vi "Tabulate TDMS Name Mapping.vi"(8 "error in":errorcluster, 11 "measurement configuration":T1={"TDMS File Path"="", "TDMS Channels"=["Chn0"], "FGEN Resource Names"=[], "TDMS Groups"=[], "FGEN Waveform Names"=[], "Waveform Sequence"=["Wfm1"], "Loops Sequence"=[], "Markers Sequence"=[]}) -> (0 "error out":errorcluster, 3 "TDMS Name Mapping":T2)   [LabVIEW 2025, in "FGEN Arb Sequence Mode.lvclass"]
uses:
  FGEN Arb Sequence Mode.lvclass
  Measurement Configuration.ctl
  67890edf-85c8-4520-b9a4-a1863d36d414.vi
  00e03d3f-0884-43fe-8b00-c6cbeff4e0a9.vi
  5d0afab6-27d8-4637-a328-ab46698b29a4.vi
  <vilib>/Utility/error.llb/Error Cluster From Error Code.vi
  <vilib>/ErrorRing/Error Ring.xnode
  FGEN Arb Sequence Mode.lvclass/FGEN Arb Sequence Mode.ctl
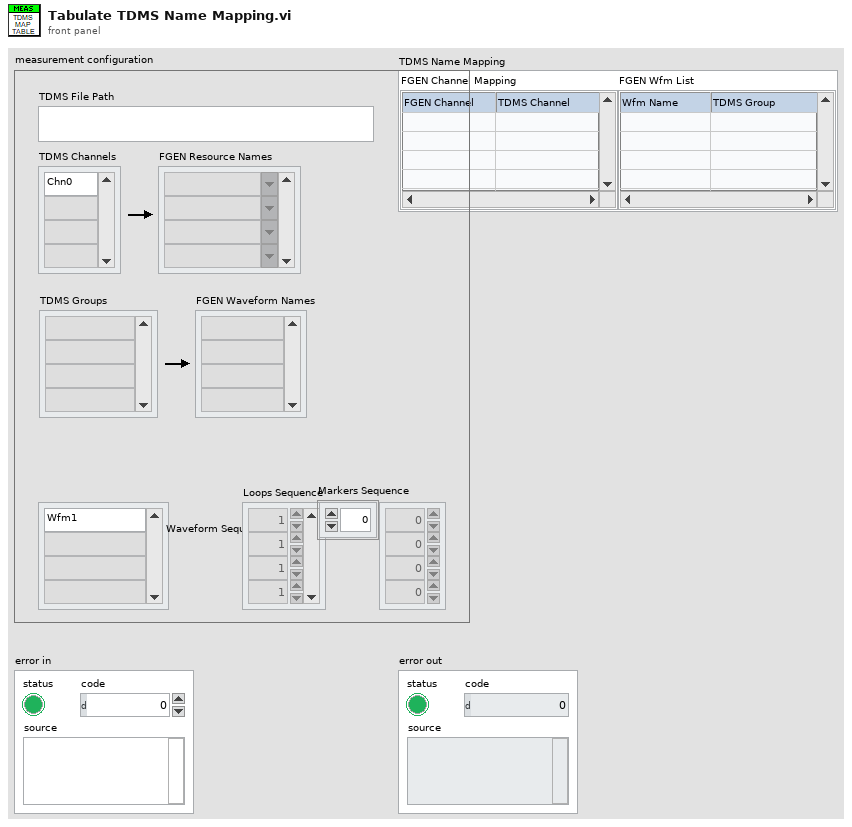
[diagram p1: front panel]
types:
  T1 = typedef "FGEN Arb Sequence Mode.lvclass/Measurement Configuration.ctl" = cluster{"TDMS File Path":string, "TDMS Channels":string[], "FGEN Resource Names":string[], "TDMS Groups":string[], "FGEN Waveform Names":string[], "Waveform Sequence":string[], "Loops Sequence":u32[], "Markers Sequence":i32[]}
  T2 = cluster{"FGEN Channel Mapping":string[][], "FGEN Wfm List":string[][]}
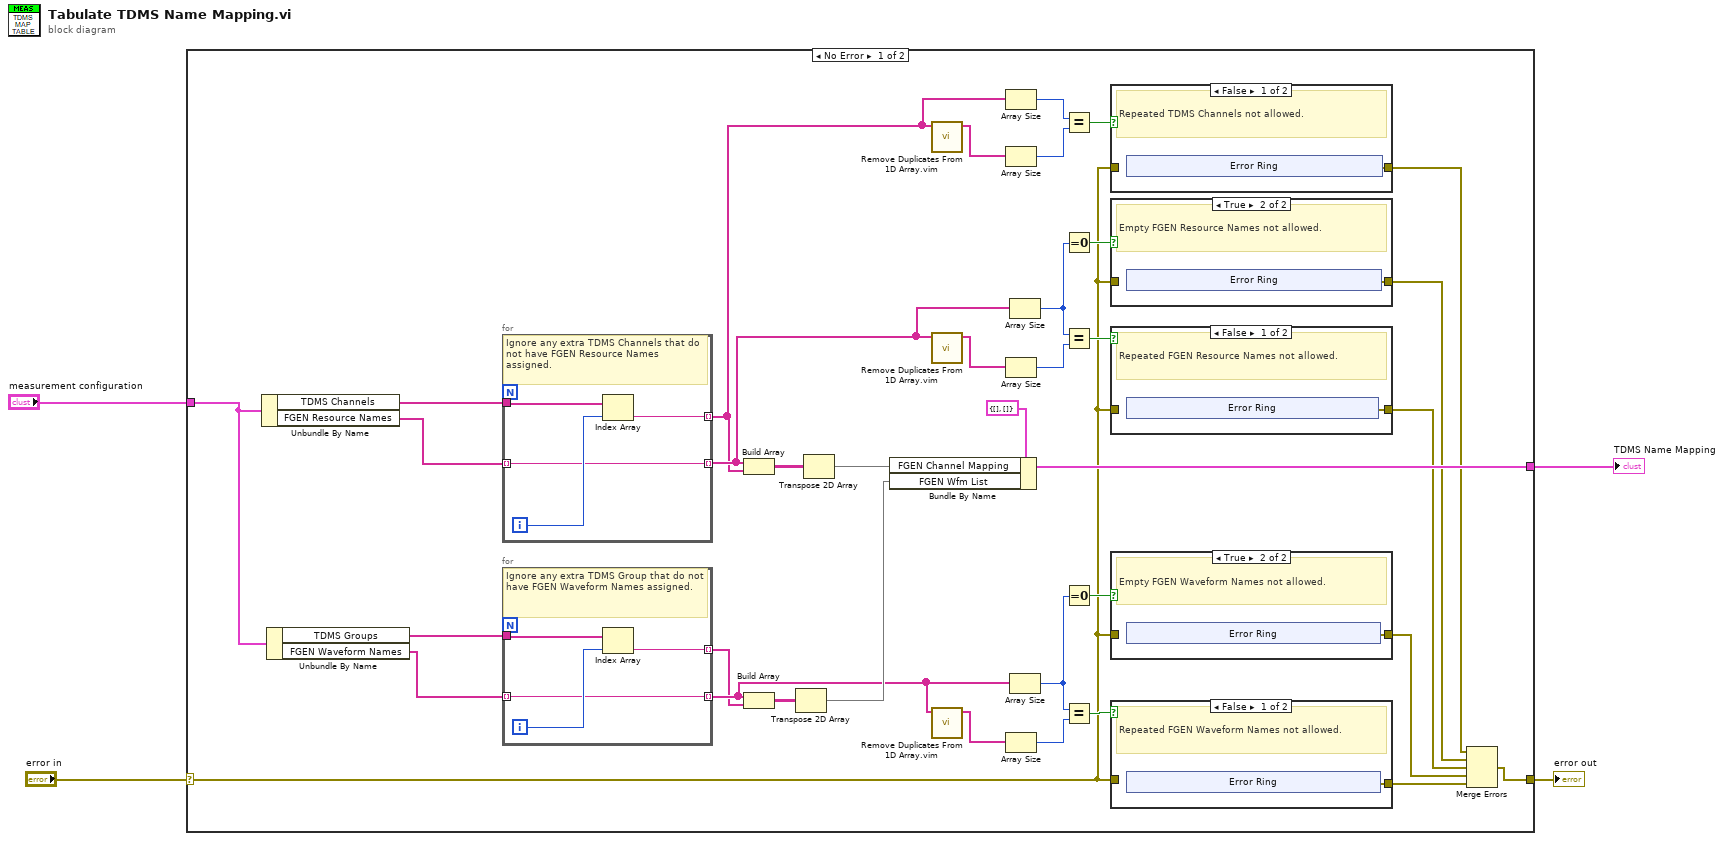
[diagram p0: block diagram]
diagram:
  n1 = case shown="No Error" "error in" {
    selector: "error in" -> [w5 w84]
    tunnel: [w26 w84] -> w3
    tunnel: "measurement configuration" -> [w40 _]
    tunnel: [w37 _] -> w1
    frame No Error {
      n2 = Unbundle By Name(w40) -> ("TDMS Channels"=w13:string[], "FGEN Resource Names"=w39:string[])
      n3 = Unbundle By Name(w40) -> ("TDMS Groups"=w9:string[], "FGEN Waveform Names"=w35:string[])
      n4 = for {
        tunnel: w39 -> [w63] mode=indexing
        tunnel: w13 -> [w65]
        tunnel: [w63] -> w29 mode=indexing
        tunnel: [w62] -> w7 mode=indexing
        i -> [w64]
        # "Ignore any extra TDMS Channels that do not have FGEN Resource Names assigned."
        n5 = Index Array(array=w65, index=w64) -> (element=w62:string)
      }
      n6 = for {
        tunnel: w35 -> [w81] mode=indexing
        tunnel: w9 -> [w83]
        tunnel: [w81] -> w22 mode=indexing
        tunnel: [w80] -> w8 mode=indexing
        i -> [w82]
        # "Ignore any extra TDMS Group that do not have FGEN Waveform Names assigned."
        n7 = Index Array(array=w83, index=w82) -> (element=w80:string)
      }
      n8 = Build Array(w29, w7) -> (w36:string[][])
      n9 = Build Array(w22, w8) -> (w34:string[][])
      n10 = Transpose 2D Array(2D array=w34) -> (transposed array=w33:string[][])
      n11 = Transpose 2D Array(2D array=w36) -> (transposed array=w32:string[][])
      n12 = Bundle By Name(cluster=T2 {"FGEN Channel Mapping"=[], "FGEN Wfm List"=[]} ("TDMS Name Mapping"), "FGEN Channel Mapping"=w32, "FGEN Wfm List"=w33) -> (w37:T2)
      n13 = call "Remove Duplicates From 1D Array.vim"("array"=w7) -> ("array with duplicates removed"=w14:string[])  [unwired: 10 in]
      n14 = call "Remove Duplicates From 1D Array.vim"("array"=w29) -> ("array with duplicates removed"=w31:string[])  [unwired: 10 in]
      n15 = call "Remove Duplicates From 1D Array.vim"("array"=w22) -> ("array with duplicates removed"=w23:string[])  [unwired: 10 in]
      n16 = Array Size(array=w7) -> (size(s)=w12:i32)
      n17 = Array Size(array=w14) -> (size(s)=w11:i32)
      n18 = Array Size(array=w31) -> (size(s)=w30:i32)
      n19 = Array Size(array=w23) -> (size(s)=w24:i32)
      n20 = Array Size(array=w29) -> (size(s)=w20:i32)
      n21 = Array Size(array=w22) -> (size(s)=w17:i32)
      n22 = Equal?(x=w12, y=w11) -> (x = y?=w10:bool)
      n23 = Equal To 0?(x=w20) -> (x = 0?=w19:bool)
      n24 = Equal?(x=w20, y=w30) -> (x = y?=w27:bool)
      n25 = Equal To 0?(x=w17) -> (x = 0?=w18:bool)
      n26 = Equal?(x=w17, y=w24) -> (x = y?=w25:bool)
      n27 = case shown="False" w10 {
        tunnel: [w41 w47] -> w6
        tunnel: w5 -> [_ w47]
        frame False {
          # "Repeated TDMS Channels not allowed."
          n28 = xnode "Error Ring"() -> ("error out"=w41:errorcluster)
        }
        frame True {
        }
      }
      n29 = case shown="True" w19 {
        tunnel: w5 -> [w48 _]
        tunnel: [w48 w49] -> w15
        frame False {
        }
        frame True {
          # "Empty FGEN Resource Names not allowed."
          n30 = xnode "Error Ring"() -> ("error out"=w49:errorcluster)
        }
      }
      n31 = case shown="False" w27 {
        tunnel: w5 -> [_ w61]
        tunnel: [w55 w61] -> w28
        frame False {
          # "Repeated FGEN Resource Names not allowed."
          n32 = xnode "Error Ring"() -> ("error out"=w55:errorcluster)
        }
        frame True {
        }
      }
      n33 = case shown="True" w18 {
        tunnel: w5 -> [w66 _]
        tunnel: [w66 w67] -> w16
        frame False {
        }
        frame True {
          # "Empty FGEN Waveform Names not allowed."
          n34 = xnode "Error Ring"() -> ("error out"=w67:errorcluster)
        }
      }
      n35 = case shown="False" w25 {
        tunnel: w5 -> [_ w79]
        tunnel: [w73 w79] -> w21
        frame False {
          # "Repeated FGEN Waveform Names not allowed."
          n36 = xnode "Error Ring"() -> ("error out"=w73:errorcluster)
        }
        frame True {
        }
      }
      n37 = Merge Errors(w6, w15, w28, w16, w21) -> (w26:errorcluster)
    }
    frame Error {
    }
  }
  "TDMS Name Mapping" <- w1
  "error out" <- w3
